vi "Find Node Url.vi"(8 "error in":errorcluster, 10 "XPath":T1(ring), 11 "DOM document":refnum<k20>) -> (0 "error out":errorcluster, 3 "Urls":path[](array[path]))   [LabVIEW 2023, in "VI Properties Editor.lvlib"]
uses:
  VI Properties Editor.lvlib
  <vilib>/xml/NI_XML.lvlib
  <resource>/objmgr/DOMUserDefRef.rc
  <vilib>/xml/Close Reference(Node).vi
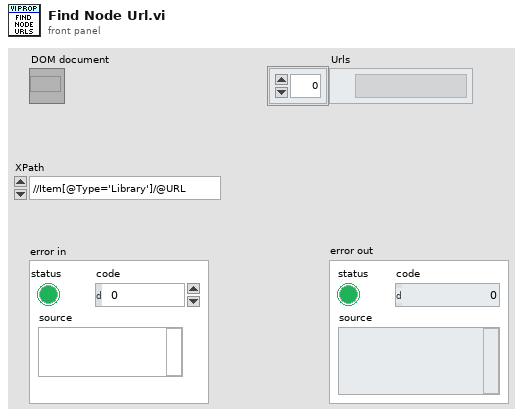
[diagram p1: front panel]
types:
  T1 = enum16{"//Item[@Type='Library']/@URL", "//Item[@Type='LVClass']/@URL"}
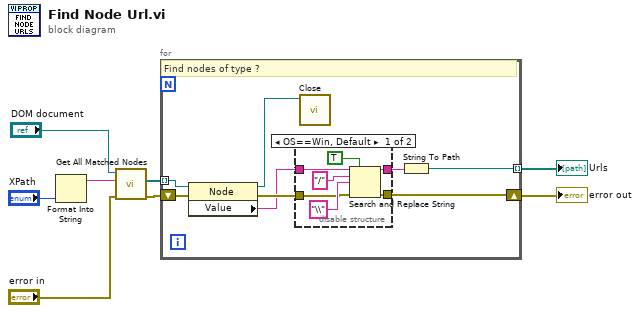
[diagram p0: block diagram]
diagram:
  n1 = Format Into String("XPath") -> (resulting string=w4:string)  [unwired: 3 in, 1 out]
  n2 = call <vilib>:"Get All Matched Nodes.vi"("error in (no error)"="error in", "XPath expression"=w4, "node in"="DOM document") -> ("error out"=w7:errorcluster, "node result array"=w8:refnum<k20>[])  [unwired: 6 in, 1 out]
  n3 = for {
    tunnel: w8 -> [w15] mode=indexing
    tunnel: [w14] -> w6 mode=indexing
    shift-right: [w13] -> w1
    shift-left: w7 -> [w16]
    # "Find nodes of type ?"
    n4 = property class="Node"(reference=w15, error in=w16) -> (reference out=w9:refnum<k20>, error out=w11:errorcluster, "Value"=w10:string)
    n5 = disable-structure shown="OS==Win, Default" {
      disable-tunnel: [w23 w25] -> w12
      disable-tunnel: w10 -> [w22 w25]
      disable-tunnel: w11 -> [w18 w24]
      disable-tunnel: [w17 w24] -> w13
      frame condition #0 (active) {
        n6 = Search and Replace String(replace all?=TRUE ("replace all? (F)"), input string=w22, search string="/", replace string="\\" ("replace string (\"\")"), error in=w18) -> (result string=w23:string, error out=w17:errorcluster)  [unwired: 3 in, 2 out]
      }
      frame condition #1 {
      }
    }
    n7 = call-poly <vilib>:"Close.vi"("node"=w9) -> ()  [unwired: 8 in, 1 out]
    n8 = String To Path(string=w12) -> (path=w14:path)
  }
  "Urls" <- w6
  "error out" <- w1
